vi "Calculadora v2.vi"() -> ()   [LabVIEW 2019]
uses:
  Control 1.ctl
  <vilib>/gmath/NI_Gmath.lvlib
panel:
  out "String 2":string
  out "String":string
  out "Numeric":dbl
  in  "Punto":bool
  in  "Button 7":bool
  in  ")":bool
  in  "(":bool
  in  "Rad":bool
  in  "ans":bool
  in  "Pi":bool
  in  "e":bool
  in  "x^1/k":bool
  in  "x^-1":bool
  in  "x!":bool
  in  "Log10":bool
  in  "x^y":bool
  in  "e ^x":bool
  in  "ln":bool
  in  "x^2":bool
  in  "x^1/2":bool
  in  "Log_x":bool
  in  "x^3":bool
  in  "x^1/3":bool
  in  "Sin":bool
  in  "Cos":bool
  in  "Tan":bool
  in  "Sinh":bool
  in  "Cosh":bool
  in  "Tanh":bool
  in  "sin^(-1)":bool
  in  "Cos^(-1)":bool
  in  "Tan^(-1)":bool
  in  "C":bool
  in  "Button =":bool
  in  "Button *":bool
  in  "Button /":bool
  in  "Button +":bool
  in  "Button 0":bool
  in  "Button -":bool
  in  "Button 9":bool
  in  "Button 8":bool
  in  "Button 6":bool
  in  "Button 5":bool
  in  "Button 4":bool
  in  "Button 3":bool
  in  "Button 2":bool
  in  "Button 1":bool
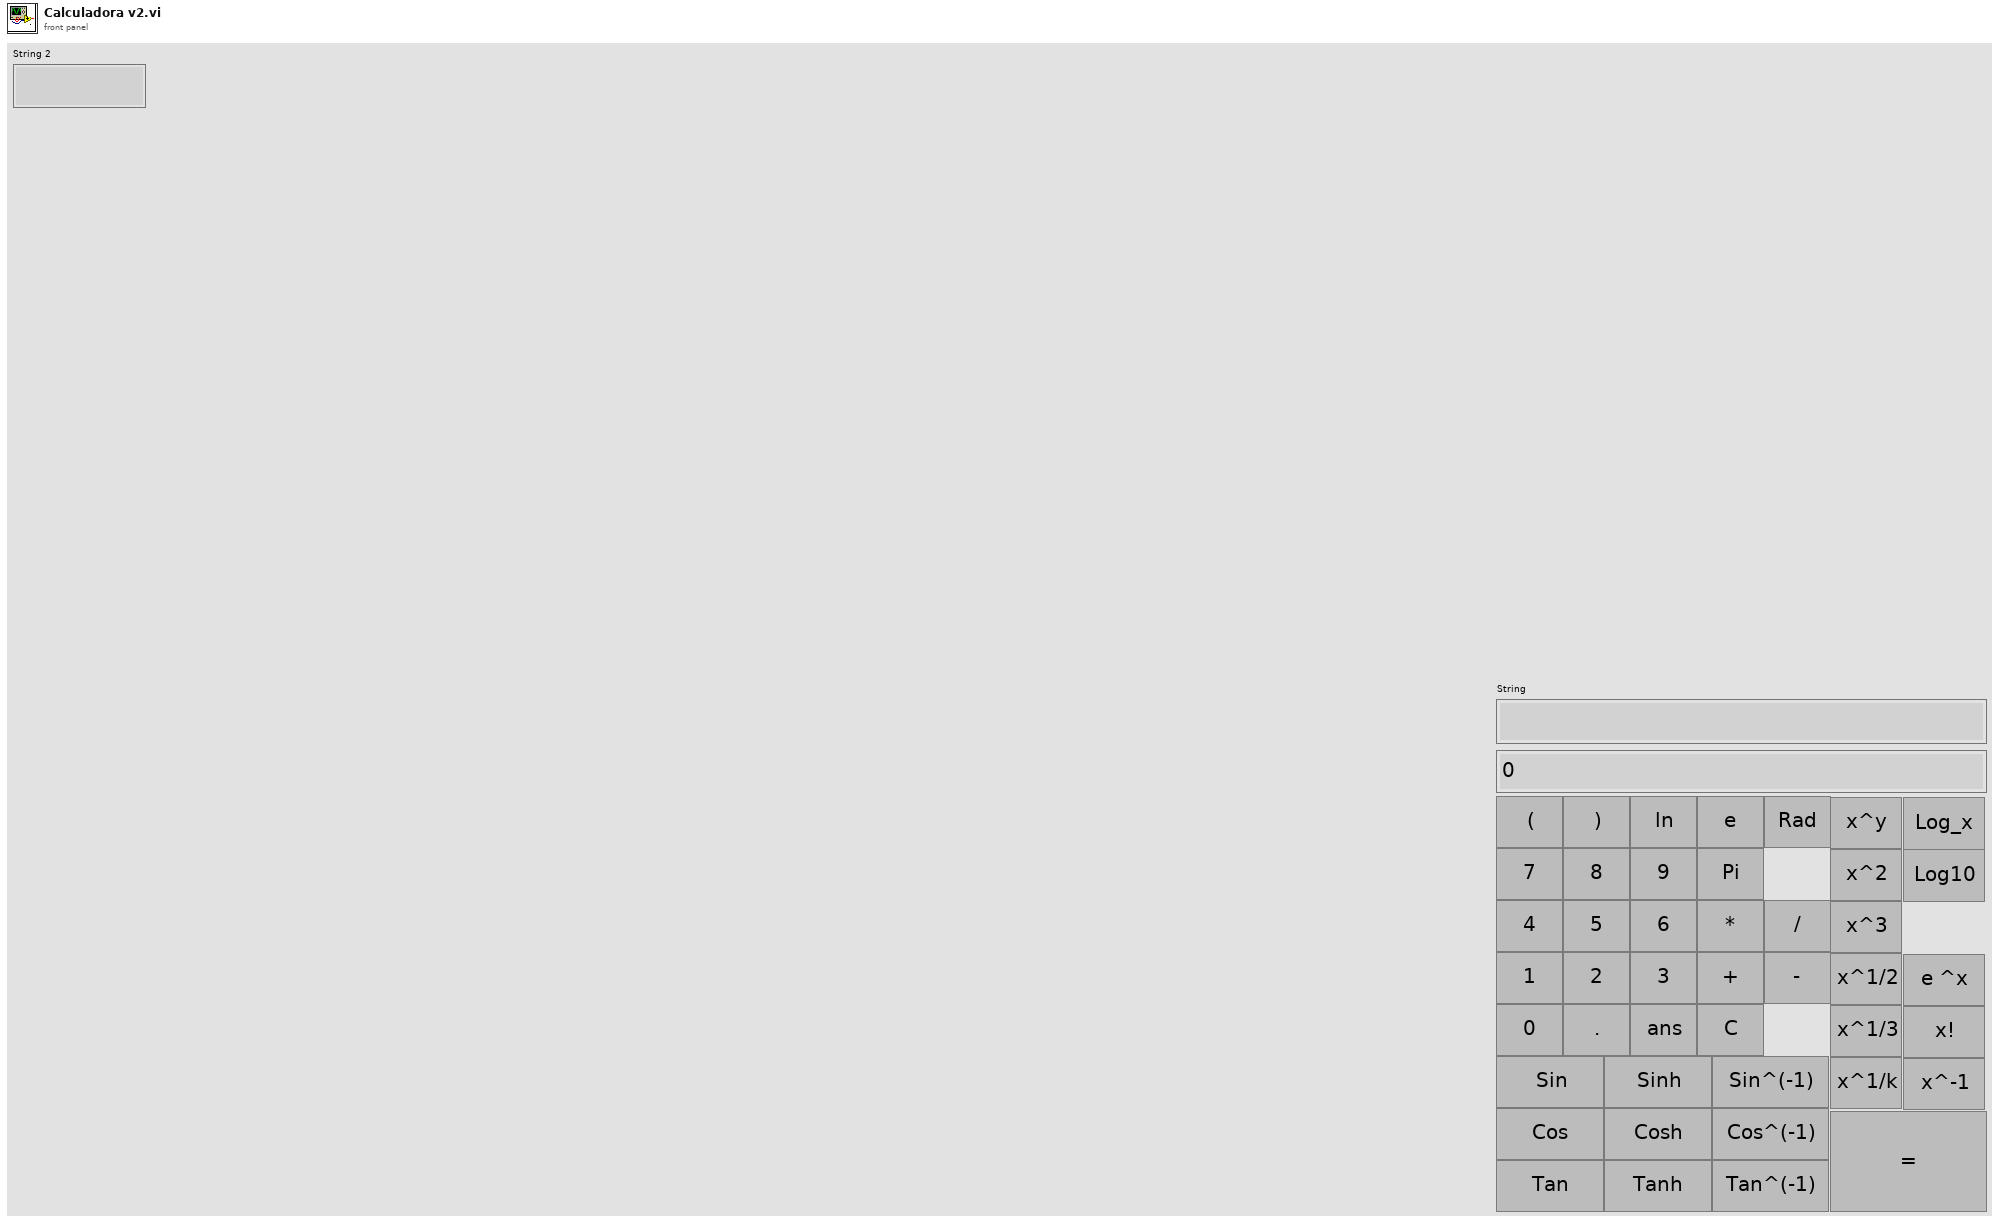
[diagram p1: front panel]
types:
  T1 = typedef "Control 1.ctl" = enum16{"x^-1", "x!", "e^x", "Log10", "Log_x", "x^1/k", "x^1/3", "x^1/2", "x^3", "x^2", "x^y", "Tan^(-1)", "Cos^(-1)", "Sin^(-1)", "Tanh", "Cosh", "Sinh", "Tan", "Cos", "Sin", "pi", "e", "ln", "+", "-", "x", "/"}
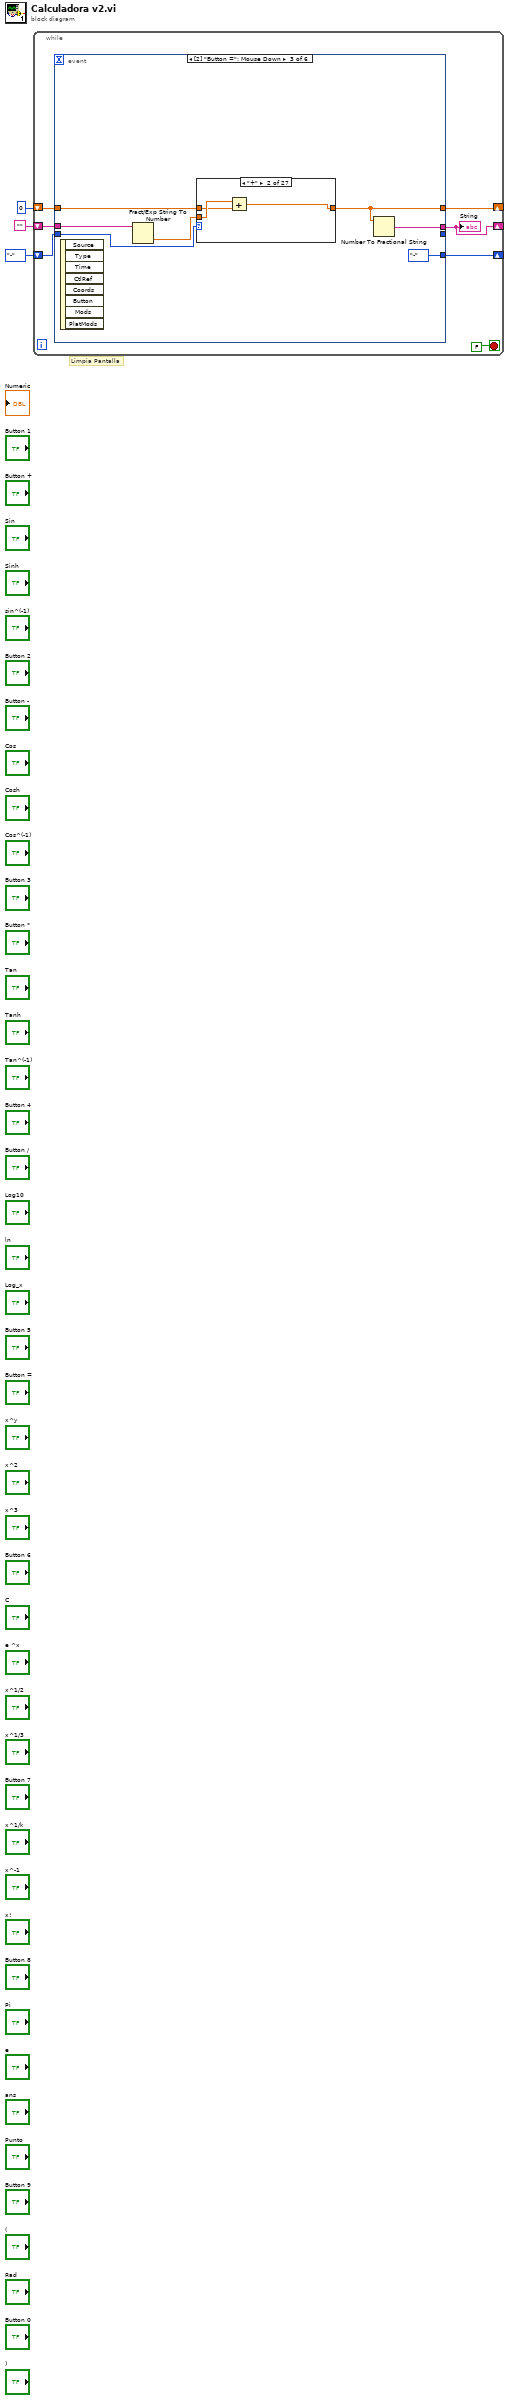
[diagram p0: block diagram]
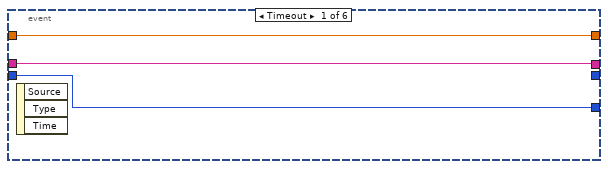
[diagram p2: hidden frame]
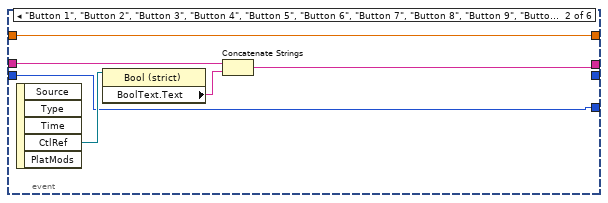
[diagram p3: hidden frame]
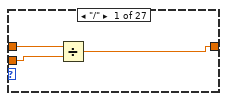
[diagram p4: hidden frame]
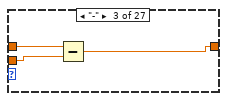
[diagram p5: hidden frame]
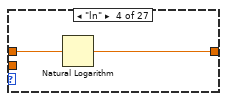
[diagram p6: hidden frame]
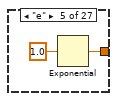
[diagram p7: hidden frame]
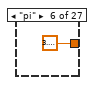
[diagram p8: hidden frame]
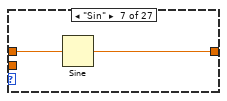
[diagram p9: hidden frame]
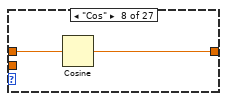
[diagram p10: hidden frame]
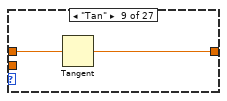
[diagram p11: hidden frame]
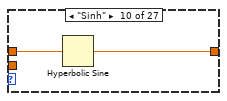
[diagram p12: hidden frame]
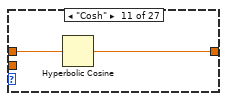
[diagram p13: hidden frame]
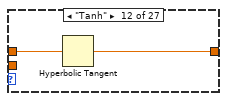
[diagram p14: hidden frame]
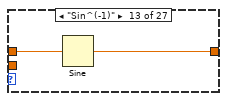
[diagram p15: hidden frame]
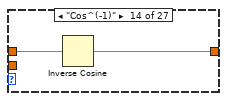
[diagram p16: hidden frame]
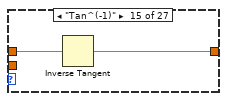
[diagram p17: hidden frame]
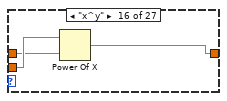
[diagram p18: hidden frame]
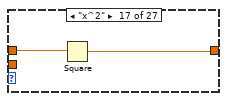
[diagram p19: hidden frame]
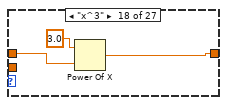
[diagram p20: hidden frame]
diagram:
  # "Limpia Pantalla"
  n1 = while {
    shift-right: [w8] -> _
    shift-left: 0 -> [w9]
    shift-right: [w6] -> _
    shift-left: Control_1."-" -> [w7]
    shift-right: [w4] -> _
    shift-left: "" -> [w5]
    stop <- FALSE stop-if-true
    n2 = event shown="[2] \"Button =\": Mouse Down" {
      selector: _ -> [_ _ _ _ _ _]
      dyn-events: _ -> [_ _ _ _ _ _]
      timeout: _ -> [_ _ _ _ _ _]
      tunnel: w9 -> [w13 w14 w22 _ _ _]
      tunnel: [w13 w14 w20 _ w100 0] -> w8
      tunnel: w7 -> [w12 w15 w23 _ w95 _]
      tunnel: [w12 w15 Control_1."-" _ w97 Control_1."+"] -> w6
      tunnel: w5 -> [w11 w18 w26 _ w101 _]
      tunnel: [w11 w16 w25 w90 "" ""] -> w4
      tunnel: [_ _ _ _ w95 _] -> _
      event Timeout {
        n3 = event-data() -> ()  [unwired: 1 in, 3 out]
      }
      event "Button 1", "Button 2", "Button 3", "Button 4", "Button 5", "Button 6", "Button 7", "Button 8", "Button 9", "Button 0", "Tan^(-1)", "Cos^(-1)", "sin^(-1)", "Tanh", "Cosh", "Sinh", "Tan", "Cos", "Sin", "x^1/3", "x^3", "Log_x", "x^1/2", "x^2", "ln", "e ^x", "x^y", "Log10", "x!", "x^-1", "x^1/k", "e", "Pi", "ans", "(", ")", "Punto": Mouse Down; "Rad": Key Down {
        n4 = event-data() -> ("CtlRef"=w19:refnum<vi>)  [unwired: 1 in, 4 out]
        n5 = property class="Bool (strict)"(reference=w19) -> ("BoolText.Text"=w17:string)  [unwired: 1 in, 2 out]
        n6 = Concatenate Strings(w18, w17) -> (w16:string)
      }
      event "Button =": Mouse Down {
        n7 = event-data() -> ()  [unwired: 1 in, 8 out]
        n8 = Fract/Exp String To Number(string=w26) -> (number=w21:dbl)  [unwired: 3 in, 1 out]
        n9 = case shown="\"+\"" w23 {
          tunnel: w21 -> [w27 w32 w34 _ _ _ _ _ _ _ _ _ _ _ _ w61 _ _ _ _ w72 w77 w78 _ _ _ _]
          tunnel: w22 -> [w28 w31 w33 w36 _ _ w41 w43 w45 w47 w49 w51 w53 w55 w57 w59 w62 w64 w67 w69 w73 w76 w79 w81 w83 w85 w87]
          tunnel: [w29 w30 w35 w37 w39 3.141592653589793 w42 w44 w46 w48 w50 w52 w54 w56 w58 w60 w63 w66 w68 w70 w74 w75 w80 w82 w84 w86 w89] -> w20
          frame "/" {
            n10 = Divide(x=w28, y=w27) -> (x/y=w29:dbl)
          }
          frame "+" {
            n11 = Add(x=w32, y=w31) -> (x+y=w30:dbl)
          }
          frame "-" {
            n12 = Subtract(x=w33, y=w34) -> (x-y=w35:dbl)
          }
          frame "ln" {
            n13 = Natural Logarithm(1:w36) -> (0:w37:dbl)
          }
          frame "e" {
            n14 = Exponential(1:1.0 ("x")) -> (0:w39:dbl)
          }
          frame "pi" {
          }
          frame "Sin" {
            n15 = Sine(x=w41) -> (sin(x)=w42:dbl)
          }
          frame "Cos" {
            n16 = Cosine(x=w43) -> (cos(x)=w44:dbl)
          }
          frame "Tan" {
            n17 = Tangent(1:w45) -> (0:w46:dbl)
          }
          frame "Sinh" {
            n18 = Hyperbolic Sine(1:w47) -> (0:w48:dbl)
          }
          frame "Cosh" {
            n19 = Hyperbolic Cosine(1:w49) -> (0:w50:dbl)
          }
          frame "Tanh" {
            n20 = Hyperbolic Tangent(1:w51) -> (0:w52:dbl)
          }
          frame "Sin^(-1)" {
            n21 = Sine(x=w53) -> (sin(x)=w54:dbl)
          }
          frame "Cos^(-1)" {
            n22 = Inverse Cosine(1:w55) -> (0:w56:dbl)
          }
          frame "Tan^(-1)" {
            n23 = Inverse Tangent(1:w57) -> (0:w58:dbl)
          }
          frame "x^y" {
            n24 = Power Of X(1:w59, 2:w61) -> (0:w60:dbl)
          }
          frame "x^2" {
            n25 = Square(x=w62) -> (x^2=w63:dbl)
          }
          frame "x^3" {
            n26 = Power Of X(1:w64, 2:3.0 ("x")) -> (0:w66:dbl)
          }
          frame "x^1/2" {
            n27 = Square Root(x=w67) -> (sqrt(x)=w68:dbl)
          }
          frame "x^1/3" {
            n28 = Y-th Root of X(1:3.0 ("x"), 2:w69) -> (0:w70:dbl)
          }
          frame "x^1/k" {
            n29 = Y-th Root of X(1:w72, 2:w73) -> (0:w74:dbl)
          }
          frame "x" {
            n30 = Multiply(x=w77, y=w76) -> (x*y=w75:dbl)
          }
          frame "Log_x" {
            n31 = Logarithm Base X(1:w78, 2:w79) -> (0:w80:dbl)
          }
          frame "Log10" {
            n32 = Logarithm Base 10(1:w81) -> (0:w82:dbl)
          }
          frame "e^x" {
            n33 = Exponential(1:w83) -> (0:w84:dbl)
          }
          frame "x!" {
            n34 = call <vilib>:"Factorial.vi"("n"=w85) -> ("n!"=w86:dbl)  [unwired: 2 in]
          }
          frame "x^-1" {
            n35 = Power Of X(1:w87, 2:-1.0 ("x")) -> (0:w89:dbl)
          }
        }
        n36 = Number To Fractional String(number=w20) -> (F-format string=w25:string)  [unwired: 3 in]
      }
      event Key Down {
        n37 = event-data() -> ("Char"=w92:i16)  [unwired: 1 in, 9 out]
        n38 = To Unsigned Byte Integer(number=w92) -> (unsigned 8bit integer=w94:u8)
        n39 = Type Cast(x=w94) -> (*(type *) &x=w93:string)  [unwired: 1 in]
        n40 = local read "String"() -> (w91:string)
        n41 = Concatenate Strings(w91, w93) -> (w90:string)
      }
      event "Button -", "Button +", "Button /", "Button *": Mouse Down {
        n42 = event-data() -> ("CtlRef"=w99:refnum<vi>)  [unwired: 1 in, 7 out]
        n43 = property class="Bool (strict)"(reference=w99) -> ("BoolText.Text"=w98:string)  [unwired: 1 in, 2 out]
        n44 = Fract/Exp String To Number(string=w101) -> (number=w100:dbl)  [unwired: 3 in, 1 out]
        n45 = case shown="\"/\"" w98 {
          tunnel: [Control_1."-" Control_1."x" Control_1."/" Control_1."+"] -> w97
          frame "-", Default {
          }
          frame "x" {
          }
          frame "/" {
          }
          frame "+" {
          }
        }
      }
      event "C": Mouse Down {
        n46 = event-data() -> ()  [unwired: 1 in, 8 out]
      }
    }
    "String" <- w4
  }
